vi "CRYAdd Step Intem Remove.vi"(8 "AddSteps":refnum<vi>, 11 "Option":string) -> ()   [LabVIEW 2013]
uses:
  CRYMainGlobal.vi
  CRYProject/CRYProject Editor Global.vi
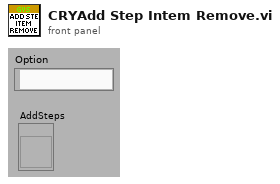
[diagram p1: front panel]
types:
  T1 = enum16{"OK", "Yes", "YesNo", "YesNoCancel", "ReplaceAppend"}
  T2 = cluster{"Content":string, "Name":string, "Level":u32, "Category":string}[]
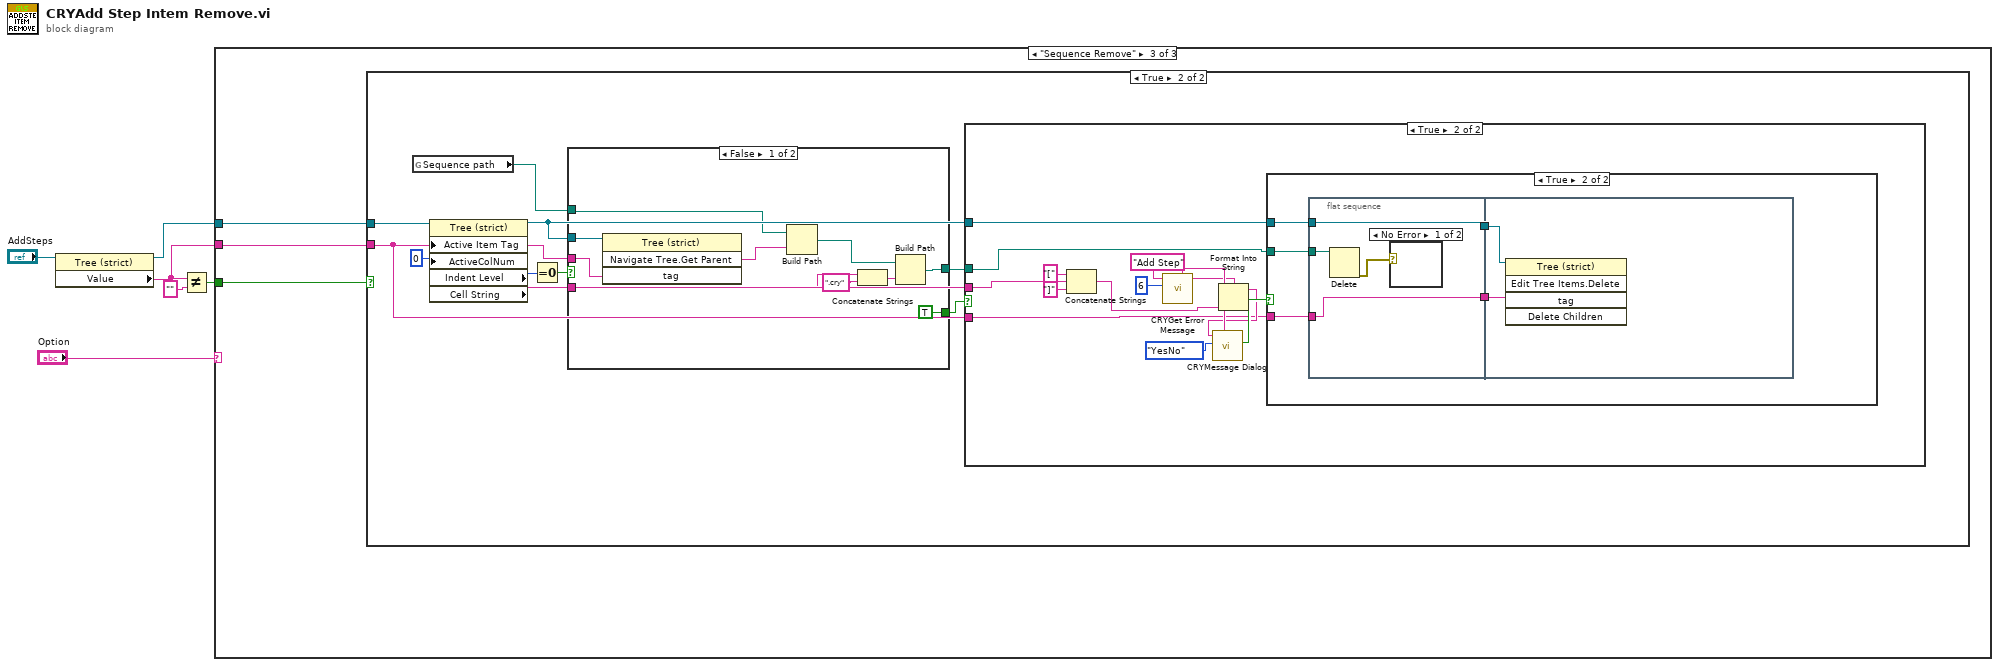
[diagram p0: block diagram]
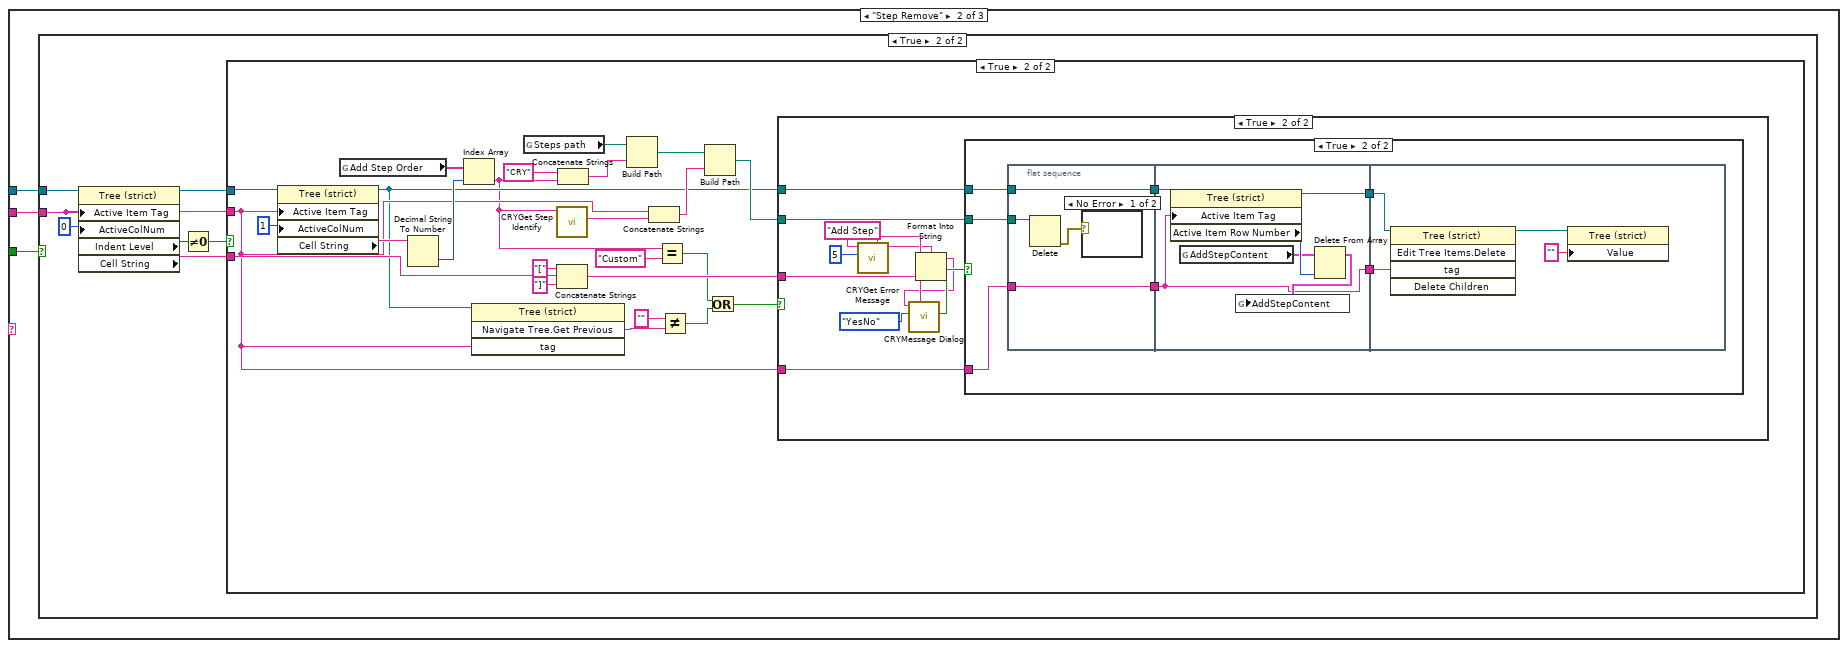
[diagram p3: hidden frame]
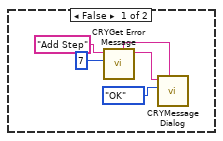
[diagram p4: hidden frame]
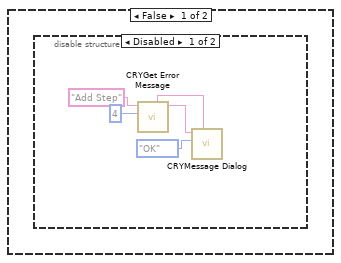
[diagram p5: hidden frame]
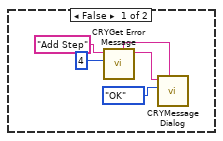
[diagram p7: hidden frame]
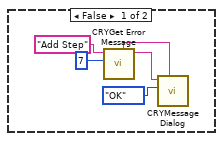
[diagram p10: hidden frame]
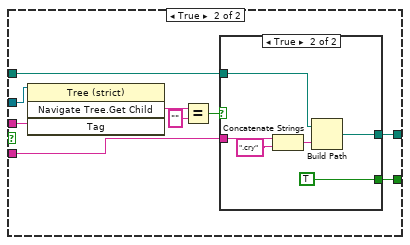
[diagram p11: hidden frame]
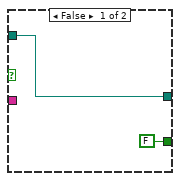
[diagram p12: hidden frame]
diagram:
  n1 = property class="Tree (strict)"(reference="AddSteps") -> (reference out=w3:refnum<vi>, "Value"=w4:string)  [unwired: 1 in, 1 out]
  n2 = Not Equal?(x=w4, y="") -> (x != y?=w5:bool)
  n3 = case shown="\"Sequence Remove\"" "Option" {
    tunnel: w5 -> [_ w9 w91]
    tunnel: w4 -> [_ w8 w90]
    tunnel: w3 -> [_ w7 w89]
    frame Default {
    }
    frame "Step Remove" {
      n4 = case shown="True" w9 {
        tunnel: w8 -> [_ w17]
        tunnel: w7 -> [_ w21]
        frame False {
          n5 = call "CRYGet Error Message.vi"("Error No"=7, "Kind"="Add Step") -> ("Message"=w11:string, "Window Title"=w12:string)  [unwired: 4 in, 4 out]
          n6 = call "CRYMessage Dialog.vi"("Window Title"=w12, "YesNoCancel"=T1."OK", "Message Content"=w11) -> ()  [unwired: 7 in, 2 out]
        }
        frame True {
          n7 = property class="Tree (strict)"(reference=w21, "Active Item Tag"=w17, "ActiveColNum"=0 ("Active Cell:Active Column Number")) -> (reference out=w18:refnum<vi>, "Indent Level"=w20:i32, "Cell String"=w15:string)  [unwired: 1 in, 1 out]
          n8 = Not Equal To 0?(x=w20) -> (x != 0?=w19:bool)
          n9 = case shown="True" w19 {
            tunnel: w18 -> [_ w36]
            tunnel: w17 -> [_ w35]
            tunnel: w15 -> [_ w44]
            frame False {
              n10 = disable-structure shown="Disabled" {
                frame Disabled {
                  n11 = call "CRYGet Error Message.vi"("Error No"=4, "Kind"="Add Step") -> ("Message"=w25:string, "Window Title"=w24:string)  [unwired: 4 in, 4 out]
                  n12 = call "CRYMessage Dialog.vi"("Window Title"=w24, "YesNoCancel"=T1."OK", "Message Content"=w25) -> ()  [unwired: 7 in, 2 out]
                }
                frame Enabled {
                }
              }
            }
            frame True {
              n13 = property class="Tree (strict)"(reference=w36, "Active Item Tag"=w35, "ActiveColNum"=1 ("Active Cell:Active Column Number")) -> (reference out=w34:refnum<vi>, "Cell String"=w38:string)  [unwired: 1 in, 1 out]
              n14 = global read "CRYMainGlobal.vi" "Add Step Order"() -> (w39:string[])
              n15 = Decimal String To Number(string=w38) -> (number=w40:i32)  [unwired: 2 in, 1 out]
              n16 = Index Array(array=w39, index=w40) -> (element=w31:string)
              n17 = invoke class="Tree (strict)" method="Navigate Tree.Get Previous"(reference=w34, "tag"=w35) -> ("Navigate Tree:Get Previous"=w33:string)  [unwired: 2 in, 3 out]
              n18 = global read "CRYMainGlobal.vi" "Steps path"() -> (w51:path)
              n19 = call "CRYGet Step Identify.vi"("Category Name In"=w31) -> ("Identfier(Regular Expression)"=w48:string)  [unwired: 3 in, 7 out]
              n20 = Concatenate Strings("[" ("string"), w44, "]" ("string")) -> (w41:string)
              n21 = Concatenate Strings("CRY" ("string"), w31) -> (w49:string)
              n22 = Build Path(base path=w51, name or relative path=w49) -> (appended path=w47:path)
              n23 = Concatenate Strings(w35, w48) -> (w46:string)
              n24 = Equal?(x=w31, y="Custom") -> (x = y?=w28:bool)
              n25 = Not Equal?(x="", y=w33) -> (x != y?=w29:bool)
              n26 = Build Path(base path=w47, name or relative path=w46) -> (appended path=w45:path)
              n27 = Or(x=w28, y=w29) -> (x .or. y?=w27:bool)
              n28 = case shown="True" w27 {
                tunnel: w45 -> [_ w67]
                tunnel: w41 -> [_ w58]
                tunnel: w34 -> [_ w59]
                tunnel: w35 -> [_ w57]
                frame False {
                  n29 = call "CRYGet Error Message.vi"("Error No"=4, "Kind"="Add Step") -> ("Message"=w55:string, "Window Title"=w54:string)  [unwired: 4 in, 4 out]
                  n30 = call "CRYMessage Dialog.vi"("Window Title"=w54, "YesNoCancel"=T1."OK", "Message Content"=w55) -> ()  [unwired: 7 in, 2 out]
                }
                frame True {
                  n31 = call "CRYGet Error Message.vi"("Error No"=5, "Kind"="Add Step") -> ("Message"=w61:string, "Window Title"=w65:string)  [unwired: 4 in, 4 out]
                  n32 = Format Into String(format string=w61, w58) -> (resulting string=w60:string)  [unwired: 2 in, 1 out]
                  n33 = call "CRYMessage Dialog.vi"("Window Title"=w65, "YesNoCancel"=T1."YesNo", "Message Content"=w60) -> ("YesNo"=w62:bool)  [unwired: 7 in, 1 out]
                  n34 = case shown="True" w62 {
                    tunnel: w67 -> [_ w74]
                    tunnel: w59 -> [_ w72]
                    tunnel: w57 -> [_ w68]
                    frame False {
                    }
                    frame True {
                      n35 = flat-sequence {
                        tunnel: w74 -> [w78]
                        tunnel: [w77] -> w73
                        tunnel: w72 -> [w77]
                        tunnel: [w76] -> w69
                        tunnel: w68 -> [w76]
                        tunnel: w73 -> [w79]
                        tunnel: [w81] -> w71
                        tunnel: [w80] -> w70
                        tunnel: w69 -> [w80]
                        tunnel: w71 -> [w88]
                        tunnel: w70 -> [w87]
                        frame #0 {
                          n36 = Delete(path (use dialog)=w78) -> (error out=w75:errorcluster)  [unwired: 4 in, 2 out]
                          n37 = case shown="No Error" w75 {
                            frame No Error {
                            }
                            frame Error {
                            }
                          }
                        }
                        frame #1 {
                          n38 = property class="Tree (strict)"(reference=w79, "Active Item Tag"=w80) -> (reference out=w81:refnum<vi>, "Active Item Row Number"=w83:i32)  [unwired: 1 in, 1 out]
                          n39 = global read "CRYProject Editor Global.vi" "AddStepContent"() -> (w82:T2)
                          n40 = Delete From Array(array=w82, index=w83) -> (array with subset deleted=w84:T2)  [unwired: 1 in, 1 out]
                          n41 = global write "CRYProject Editor Global.vi" "AddStepContent"(w84) -> ()
                        }
                        frame #2 {
                          n42 = invoke class="Tree (strict)" method="Edit Tree Items.Delete"(reference=w88, "tag"=w87) -> (reference out=w86:refnum<vi>)  [unwired: 3 in, 4 out]
                          n43 = property class="Tree (strict)"(reference=w86, "Value"="") -> ()  [unwired: 1 in, 2 out]
                        }
                      }
                    }
                  }
                }
              }
            }
          }
        }
      }
    }
    frame "Sequence Remove" {
      n44 = case shown="True" w91 {
        tunnel: w90 -> [_ w101]
        tunnel: w89 -> [_ w106]
        frame False {
          n45 = call "CRYGet Error Message.vi"("Error No"=7, "Kind"="Add Step") -> ("Message"=w93:string, "Window Title"=w94:string)  [unwired: 4 in, 4 out]
          n46 = call "CRYMessage Dialog.vi"("Window Title"=w94, "YesNoCancel"=T1."OK", "Message Content"=w93) -> ()  [unwired: 7 in, 2 out]
        }
        frame True {
          n47 = global read "CRYMainGlobal.vi" "Sequence path"() -> (w99:path)
          n48 = property class="Tree (strict)"(reference=w106, "Active Item Tag"=w101, "ActiveColNum"=0 ("Active Cell:Active Column Number")) -> (reference out=w102:refnum<vi>, "Indent Level"=w104:i32, "Cell String"=w100:string)  [unwired: 1 in, 1 out]
          n49 = Equal To 0?(x=w104) -> (x = 0?=w103:bool)
          n50 = case shown="False" w103 {
            tunnel: w100 -> [w114 w123]
            tunnel: [w113 w125] -> w97
            tunnel: w99 -> [w110 w124]
            tunnel: w102 -> [w112 w121]
            tunnel: w101 -> [w111 w120]
            tunnel: [TRUE ("x = 0?") w122] -> w98
            frame False {
              n51 = invoke class="Tree (strict)" method="Navigate Tree.Get Parent"(reference=w112, "tag"=w111) -> ("Navigate Tree:Get Parent"=w109:string)  [unwired: 2 in, 3 out]
              n52 = Build Path(base path=w110, name or relative path=w109) -> (appended path=w108:path)
              n53 = Concatenate Strings(w114, ".cry" ("string")) -> (w116:string)
              n54 = Build Path(base path=w108, name or relative path=w116) -> (appended path=w113:path)
            }
            frame True {
              n55 = invoke class="Tree (strict)" method="Navigate Tree.Get Child"(reference=w121, "Tag"=w120) -> ("Navigate Tree:Get Child"=w119:string)  [unwired: 2 in, 3 out]
              n56 = Equal?(x=w119, y="") -> (x = y?=w117:bool)
              n57 = case shown="True" w117 {
                tunnel: [w127 w133] -> w125
                tunnel: w124 -> [w127 w130]
                tunnel: w123 -> [_ w129]
                tunnel: [FALSE ("x = 0?") TRUE ("x = 0?")] -> w122
                frame False {
                }
                frame True {
                  n58 = Concatenate Strings(w129, ".cry" ("string")) -> (w132:string)
                  n59 = Build Path(base path=w130, name or relative path=w132) -> (appended path=w133:path)
                }
              }
            }
          }
          n60 = case shown="True" w98 {
            tunnel: w102 -> [_ w140]
            tunnel: w101 -> [_ w139]
            tunnel: w100 -> [_ w138]
            tunnel: w97 -> [_ w134]
            frame False {
            }
            frame True {
              n61 = Concatenate Strings("[" ("string"), w138, "]" ("string")) -> (w135:string)
              n62 = call "CRYGet Error Message.vi"("Error No"=6, "Kind"="Add Step") -> ("Message"=w142:string, "Window Title"=w146:string)  [unwired: 4 in, 4 out]
              n63 = Format Into String(format string=w142, w135) -> (resulting string=w141:string)  [unwired: 2 in, 1 out]
              n64 = call "CRYMessage Dialog.vi"("Window Title"=w146, "YesNoCancel"=T1."YesNo", "Message Content"=w141) -> ("YesNo"=w143:bool)  [unwired: 7 in, 1 out]
              n65 = case shown="True" w143 {
                tunnel: w134 -> [_ w152]
                tunnel: w140 -> [_ w151]
                tunnel: w139 -> [_ w148]
                frame False {
                }
                frame True {
                  n66 = flat-sequence {
                    tunnel: [w155] -> w150
                    tunnel: [w156] -> w149
                    tunnel: w148 -> [w156]
                    tunnel: w151 -> [w155]
                    tunnel: w152 -> [w154]
                    tunnel: w150 -> [w158]
                    tunnel: w149 -> [w157]
                    frame #0 {
                      n67 = Delete(path (use dialog)=w154) -> (error out=w153:errorcluster)  [unwired: 4 in, 2 out]
                      n68 = case shown="No Error" w153 {
                        frame No Error {
                        }
                        frame Error {
                        }
                      }
                    }
                    frame #1 {
                      n69 = invoke class="Tree (strict)" method="Edit Tree Items.Delete"(reference=w158, "tag"=w157) -> ()  [unwired: 3 in, 5 out]
                    }
                  }
                }
              }
            }
          }
        }
      }
    }
  }
